vi "配置对话框.vi"() -> ()   [LabVIEW 2016, in "opSignIn.lvlib"]
uses:
  opSignIn.lvlib
panel:
  out "sync":bool
  in  "自动获取MN":bool=TRUE
  in  "保存":bool
  in  "userType":string="equip"
  in  "MN":string="STDTEST001"
  in  "scope":string="read"
  in  "password":string="59315200"
  in  "grantType":string="password"
  in  "clientSecret":string="test_secret"
  in  "clientId":string="test_client"
  in  "url":string="http://dev.watersystem.com.cn:36091"
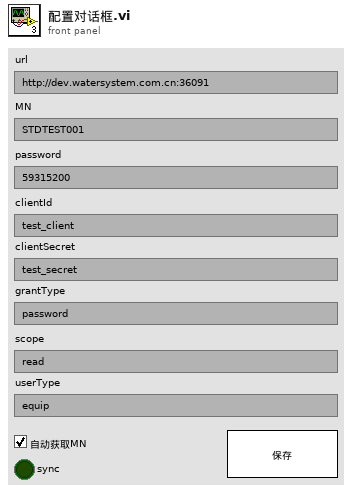
[diagram p1: front panel]
types:
  T1 = cluster{"url":string, "loginTokenRequest":cluster{"clientId":string, "clientSecret":string, "grantType":string, "password":string, "scope":string, "userName":string, "userType":string}, "自动获取MN":bool}
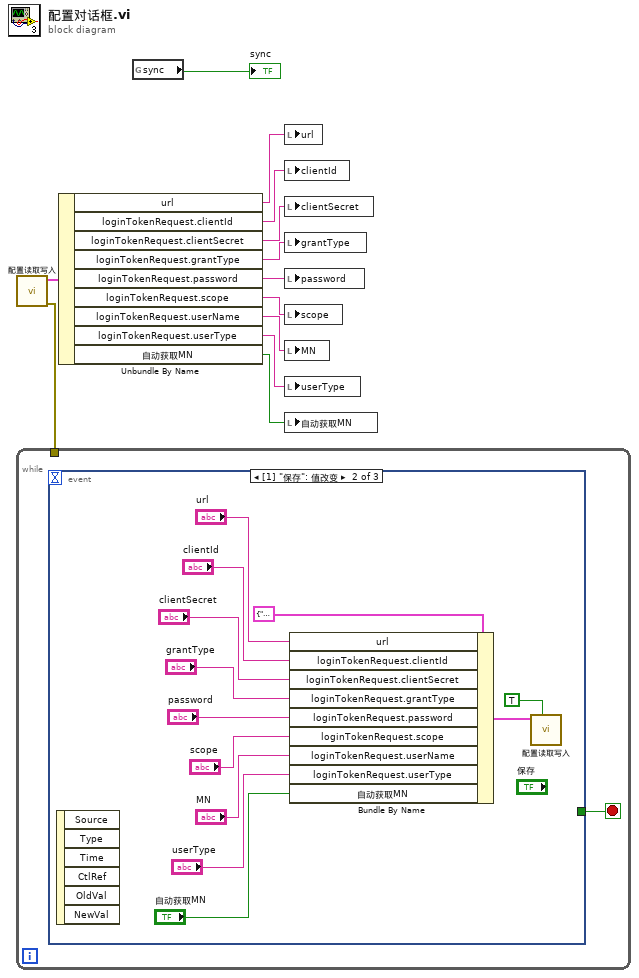
[diagram p0: block diagram]
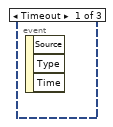
[diagram p2: hidden frame]
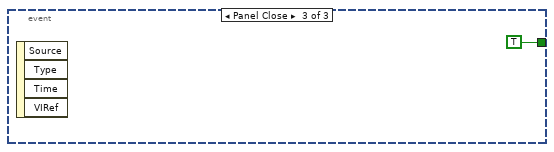
[diagram p3: hidden frame]
diagram:
  n1 = call "配置读取写入.vi"() -> ("error out"=w2:errorcluster, "配置输出"=w12:T1)  [unwired: 10 in]
  n2 = while {
    tunnel: w2 -> [_]
    stop <- w13 stop-if-true
    n3 = event shown="[1] \"保存\": 值改变" {
      selector: _ -> [_ _ _]
      dyn-events: _ -> [_ _ _]
      timeout: _ -> [_ _ _]
      tunnel: [_ _ TRUE] -> w13
      event Timeout {
        n4 = event-data() -> ()  [unwired: 1 in, 3 out]
      }
      event "保存": Value Change {
        n5 = event-data() -> ()  [unwired: 1 in, 6 out]
        n6 = Bundle By Name(cluster=T1 {"url"="http://data.watersystem.com.cn:50040", "loginTokenRequest"={"clientId"="wqms_equip", "clientSecret"="2gJxw%vZkRGX8K7Se$^q", "grantType"="password", "password"="123456", "scope"="read", "userName"="equipapi", "userType"="equip"}, "自动获取MN"=TRUE} ("配置"), "url"="url", "loginTokenRequest.clientId"="clientId", "loginTokenRequest.clientSecret"="clientSecret", "loginTokenRequest.grantType"="grantType", "loginTokenRequest.password"="password", "loginTokenRequest.scope"="scope", "loginTokenRequest.userName"="MN", "loginTokenRequest.userType"="userType", "自动获取MN"="自动获取MN") -> (w14:T1)
        n7 = call "配置读取写入.vi"("write"=TRUE, "配置"=w14) -> ()  [unwired: 8 in, 2 out]
      }
      event Panel Close {
        n8 = event-data() -> ()  [unwired: 1 in, 4 out]
      }
    }
  }
  n9 = Unbundle By Name(w12) -> ("url"=w11:string, "loginTokenRequest.clientId"=w10:string, "loginTokenRequest.clientSecret"=w9:string, "loginTokenRequest.grantType"=w8:string, "loginTokenRequest.password"=w7:string, "loginTokenRequest.scope"=w6:string, "loginTokenRequest.userName"=w5:string, "loginTokenRequest.userType"=w4:string, "自动获取MN"=w3:bool)
  n10 = global read "工况数据接口全局.vi" "sync"() -> (→"sync":bool)
  n11 = local write "url"(w11) -> ()
  n12 = local write "clientId"(w10) -> ()
  n13 = local write "clientSecret"(w9) -> ()
  n14 = local write "grantType"(w8) -> ()
  n15 = local write "password"(w7) -> ()
  n16 = local write "scope"(w6) -> ()
  n17 = local write "MN"(w5) -> ()
  n18 = local write "userType"(w4) -> ()
  n19 = local write "自动获取MN"(w3) -> ()
